vi "FunctMgr.Push Return Info.vi"(8 "error in (no error)":errorcluster, 10 "Ret Info":variant, 11 "FunctMgr in":refnum<class "FunctMgr.lvclass">) -> (0 "error out":errorcluster, 1 "Valid Msg":bool, 2 "Ret ID":string, 3 "FunctMgr out":refnum<class "FunctMgr.lvclass">)   [LabVIEW 2024, in "FunctMgr.lvclass"]
uses:
  FunctMgr.lvclass
  <vilib>/KATE/Queues/Q.Msg Return Info.ctl
  <vilib>/KATE/Queues/Q.Element.ctl
  <vilib>/KATE/SeqMgr/SeqMgr.Ret Msg Info.ctl
  FunctMgr.lvclass/FunctMgr.ctl
  <vilib>/KATE/Queues/Queue Utils.lvlib
  <vilib>/KATE/SeqMgr/SeqMgr.lvlib
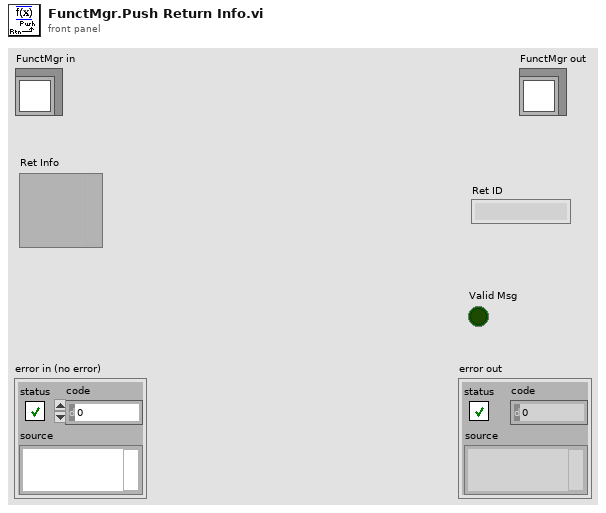
[diagram p1: front panel]
types:
  T1 = typedef "KATE_Lib.lvlib/Queue Utils.lvlib/Q.Msg Return Info.ctl" = cluster{"Ret Q":refnum<queue>, "Ret Msg":T2, "SeqNum":i32}
  T2 = typedef "KATE_Lib.lvlib/Queue Utils.lvlib/Q.Element.ctl" = cluster{"Cmd":string, "Sub":string, "Data1":variant, "Data2":variant}
  T3 = typedef "KATE_Lib.lvlib/SeqMgr.lvlib/SeqMgr.Ret Msg Info.ctl" = cluster{"ID":string, "Data":variant, "Ret Req":T1, "Error":errorcluster}
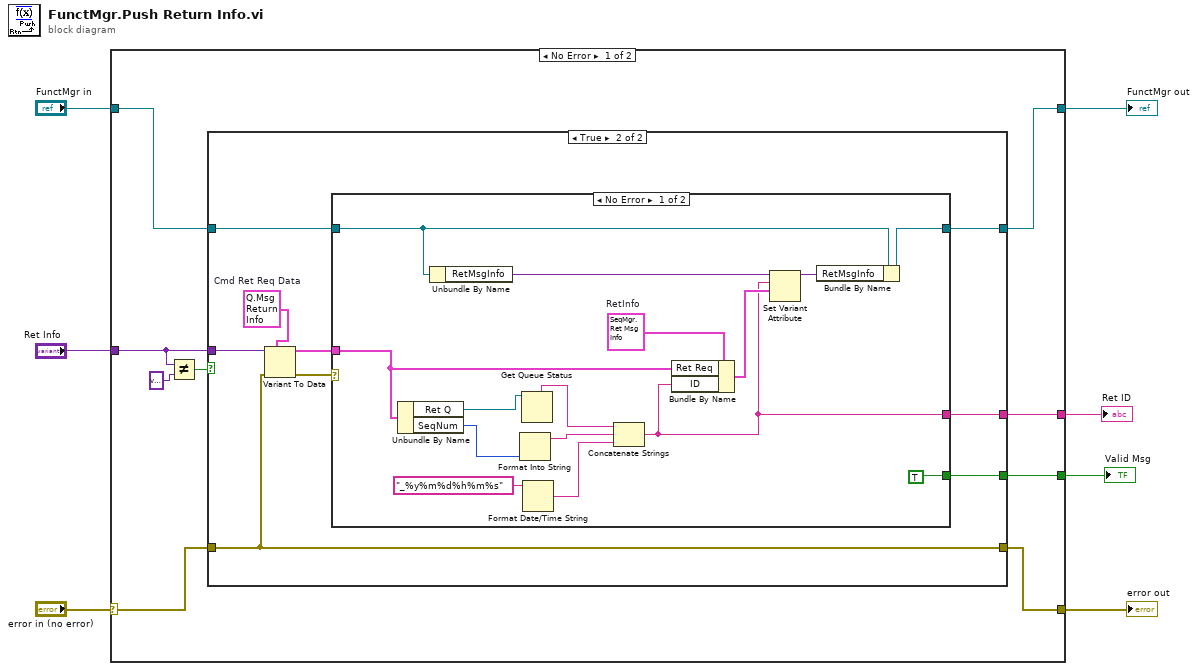
[diagram p0: block diagram]
diagram:
  n1 = case shown="No Error" "error in (no error)" {
    selector: "error in (no error)" -> [w8 w45]
    tunnel: [w9 w45] -> w6
    tunnel: [w10 w44] -> w4
    tunnel: "FunctMgr in" -> [w11 w44]
    tunnel: [w14 _] -> w3
    tunnel: [w13 _] -> w2
    tunnel: "Ret Info" -> [w12 _]
    frame No Error {
      n2 = Not Equal?(x=w12, y=variant) -> (x != y?=w16:bool)
      n3 = case shown="True" w16 {
        tunnel: [w17 w27] -> w9
        tunnel: w11 -> [w18 w26]
        tunnel: [w18 w25] -> w10
        tunnel: w12 -> [_ w24]
        tunnel: [_ w21] -> w14
        tunnel: w8 -> [w17 w27]
        tunnel: [_ w19] -> w13
        frame False {
          # "Ret info is empty - do nothing"
        }
        frame True {
          w23 = T1 {"Ret Q"=refnum, "Ret Msg"={"Cmd"="", "Sub"="", "Data1"=variant, "Data2"=variant}, "SeqNum"=0}  # Cmd Ret Req Data
          n4 = Variant To Data(error in=w27, type=w23, Variant=w24) -> (data=w22:T1, error out=w20:errorcluster)
          n5 = case shown="No Error" w20 {
            tunnel: [w42 w43] -> w25
            tunnel: w26 -> [w41 w43]
            tunnel: [w28 _] -> w21
            tunnel: w22 -> [w30 _]
            tunnel: [TRUE _] -> w19
            frame No Error {
              w31 = T3 {"ID"="", "Data"=variant, "Ret Req"={"Ret Q"=refnum, "Ret Msg"={"Cmd"="", "Sub"="", "Data1"=variant, "Data2"=variant}, "SeqNum"=0}, "Error"={"status"=FALSE, "code"=0, "source"=""}}  # RetInfo
              n6 = Unbundle By Name(w30) -> ("Ret Q"=w36:refnum<queue>, "SeqNum"=w37:i32)
              n7 = Unbundle By Name(w41) -> ("RetMsgInfo"=w39:variant)
              n8 = Format Into String(w37) -> (resulting string=w34:string)  [unwired: 3 in, 1 out]
              n9 = Get Queue Status(queue=w36) -> (queue name=w35:string)  [unwired: 2 in, 7 out]
              n10 = Format Date/Time String(time format string (%c)="_%y%m%d%h%m%s") -> (date/time string=w33:string)  [unwired: 2 in]
              n11 = Concatenate Strings(w35, w34, w33) -> (w28:string)
              n12 = Bundle By Name(cluster=w31, "Ret Req"=w30, "ID"=w28) -> (w29:T3)
              n13 = Set Variant Attribute(Variant=w39, name=w28, value=w29) -> (Variant out=w38:variant)  [unwired: 1 in, 2 out]
              n14 = Bundle By Name(cluster=w41, "RetMsgInfo"=w38) -> (w42:refnum<class "FunctMgr.lvclass">)
            }
            frame Error {
              # "If invalid Cmd Msg Info then do nothing"
            }
          }
        }
      }
    }
    frame Error {
    }
  }
  "error out" <- w6
  "FunctMgr out" <- w4
  "Ret ID" <- w3
  "Valid Msg" <- w2
